vi "ziSetValueDoubleArray.vi"(3 "Error In":errorcluster, 4 "Values":dbl[](array[numeric]), 5 "Paths":string[](array[string]), 6 "Handle In":T1 {"Handle" format="0x%08x"; "Conn" format="0x%08x"}) -> (0 "Error Out":errorcluster, 2 "Handle Out":T1 {"Handle" format="0x%08x"; "Conn" format="0x%08x"})   [LabVIEW 2009, in "Zurich Instruments LabOne.lvlib"]
doc: "This vi sets values to the nodes specified in Path to Value. More than one node can be set if a wildcard is used in Path. The i-th element of Paths receives the i-th value of Values."
uses:
  <instrlib>/Zurich Instruments LabOne/Zurich Instruments LabOne.lvlib
  <instrlib>/Zurich Instruments LabOne/Public/ziTypeHandle.ctl
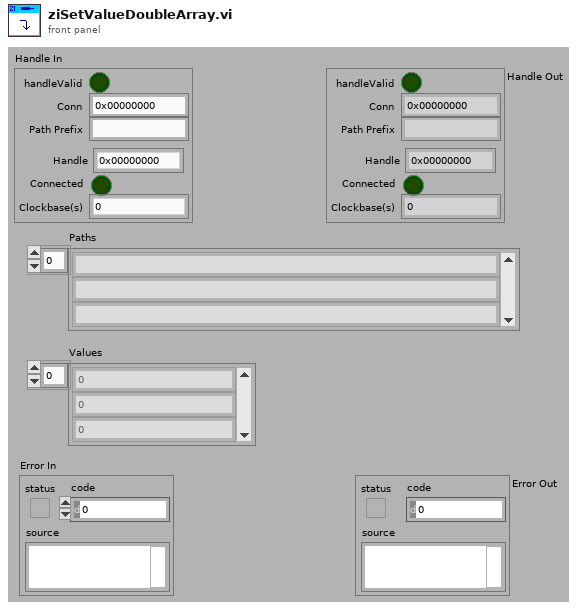
[diagram p1: front panel]
types:
  T1 = typedef "Zurich Instruments LabOne.lvlib/ziTypeHandle.ctl" = cluster{"handleValid":bool, "Conn":u64, "Path Prefix":string, "Handle":u64, "Connected":bool, "Clockbase(s)":dbl}
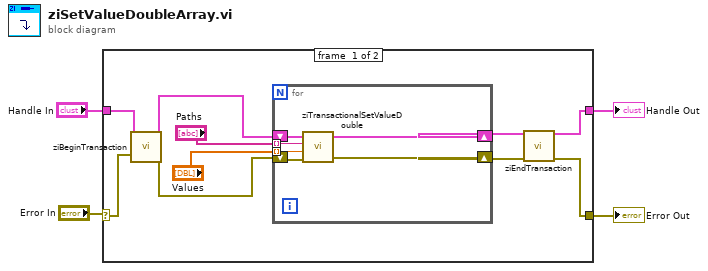
[diagram p0: block diagram]
diagram:
  n1 = case shown="No Error" "Error In" {
    selector: "Error In" -> [w6 w22]
    tunnel: [w9 w22] -> w4
    tunnel: [w10 w21] -> w3
    tunnel: "Handle In" -> [w8 w21]
    frame #0 {
      n2 = call <instrlib>:"ziBeginTransaction.vi"("Handle In"=w8, "Error In"=w6) -> ("Handle Out"=w7:T1, "Error Out"=w5:errorcluster)  [unwired: 12 in]
      n3 = for {
        tunnel: "Paths" -> [w20] mode=indexing
        tunnel: "Values" -> [w19] mode=indexing
        shift-right: [w17] -> w12
        shift-left: w5 -> [w18]
        shift-right: [w16] -> w11
        shift-left: w7 -> [w15]
        n4 = call <instrlib>:"ziTransactionalSetValueDouble.vi"("Error In"=w18, "Value"=w19, "Path"=w20, "Handle In"=w15) -> ("Error Out"=w17:errorcluster, "Handle Out"=w16:T1)  [unwired: 1 in]
      }
      n5 = call <instrlib>:"ziEndTransaction.vi"("Handle In"=w11, "Error In"=w12) -> ("Handle Out"=w10:T1, "Error Out"=w9:errorcluster)  [unwired: 12 in]
    }
    frame #1 {
    }
  }
  "Error Out" <- w4
  "Handle Out" <- w3
